vi "DB5000.W写.vi"(0 "gInitialSIEMENSS7 In":refnum<k24>, 1 "地址数组":string[](array[string])=["DB5000.228"], 2 "value":u16, 5 "error in (no error)":errorcluster caption="错误输入（无错误）") -> (14 "gInitialSIEMENSS7 Out":refnum<k24>, 19 "error out":errorcluster caption="错误输出")   [LabVIEW 2017]
panel:
  in  "一致性检测结果 2":u16
  out "数组 2":string[](array[string])
  # "DB5000,W228"
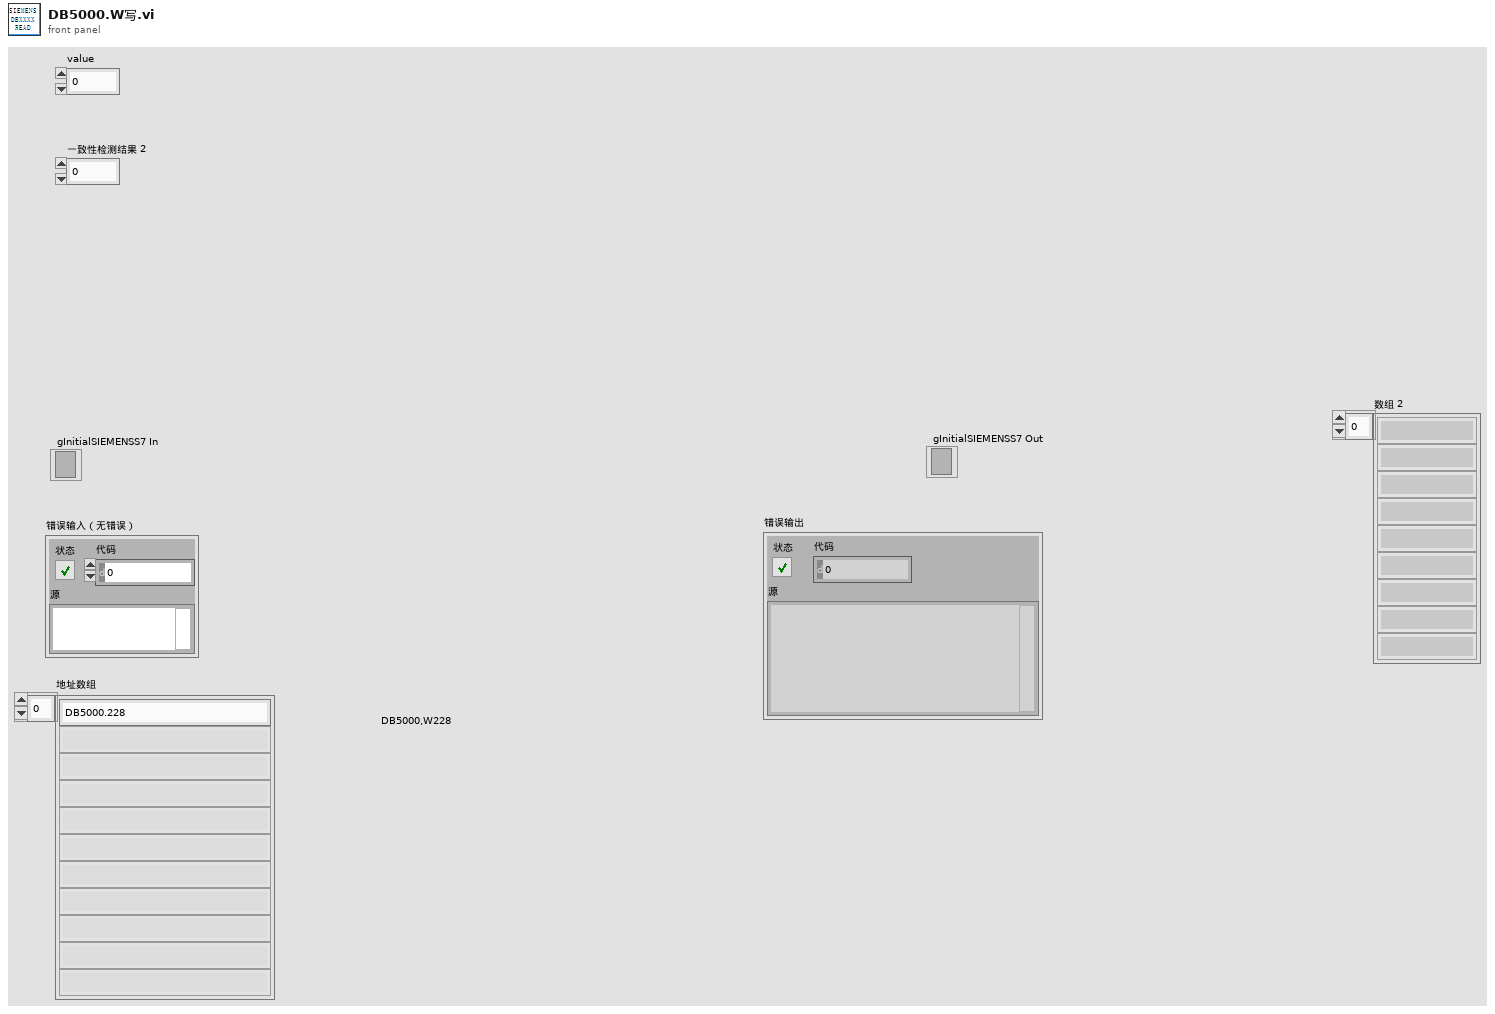
[diagram p1: front panel]
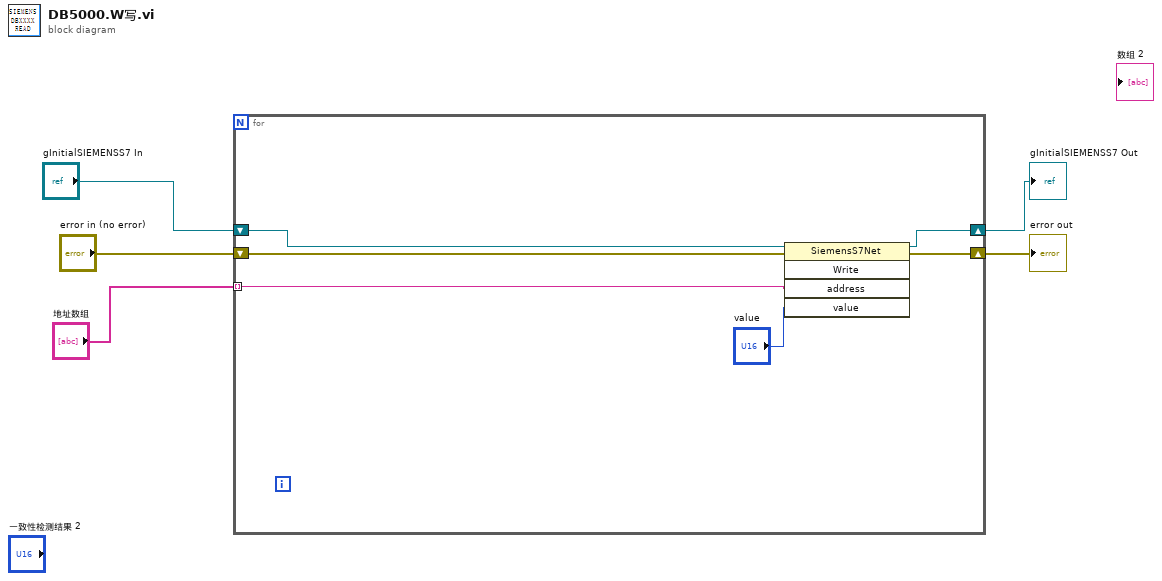
[diagram p0: block diagram]
diagram:
  n1 = for {
    tunnel: "地址数组" -> [w6] mode=indexing
    shift-right: [w8] -> w3
    shift-left: "error in (no error)" -> [w8]
    shift-right: [w10] -> w4
    shift-left: "gInitialSIEMENSS7 In" -> [w7]
    n2 = invoke class="SiemensS7Net" method="Write"(reference=w7, "address"=w6, "value"="value") -> (reference out=w10:refnum<k24>)  [unwired: 2 in, 4 out]
  }
  "gInitialSIEMENSS7 Out" <- w4
  "error out" <- w3
